vi "ReadFromFIFO.vi"(10 "stop":bool) -> (2 "This is what I told you!":string)   [LabVIEW 2011]
doc: "Elizabeth Mahon\nBased off of example from LabView and IGVC 3.2.1 Read VectorNav.\nReads data from compass sensor on port 1 of the serial module from a FIFO and outputs it as a string.\nStarts as waiting, then when it reads $ (first element of compass string) starts reading and adds everything it reads together until it reaches *ss (where ss can be anything, the \"two digit checksum\"), and then stops and outputs the string.\nOnly reads the string once - must be run in a while loop for multiple readings.\nJust shuts down if it has an error. In the future, we might want to output if it has an error."
uses:
  <vilib>/FPGAPlugInAG/cRIO-9113/niLvFpga_Open_cRIO-9113.vi
  <vilib>/rvi/interface/common/dynamic/niFpgaDynamicAddResources.vi
  <vilib>/Utility/error.llb/Error Cluster From Error Code.vi
  <vilib>/rvi/errors/niLvFpgaAdjustHostInterfaceError.vi
  <vilib>/FPGAPlugInAG/Dynamic/niLvFpga_Close_Dynamic.vi
  <vilib>/rvi/interface/nirviOpenFPGA/nirviOpenFPGA.xnode
  FPGA Bitfiles/SailBot_FPGATarget_WriteToFIFO_EBA82491.lvbitx
  1A-FPGA/1A Code/WriteToFIFO.vi
  <vilib>/rvi/interface/nirviMethod/nirviMethod.xnode
  <vilib>/rvi/interface/nirviCloseFPGA/nirviCloseFPGA.xnode
  <vilib>/FPGAPlugInAG/Dynamic/niLvFpga_ReadFifo_Dynamic.vi
  <vilib>/rvi/errors/niLvFpgaMergeErrorWithErrorCode.vi
panel:
  out "Current Status":enum16{"Waiting", "Reading", "Time Out!"}(ring)
  out "Data":i16[](array[numeric])
  in  "Status":enum16{"Waiting", "Reading", "Time Out!"}(ring)
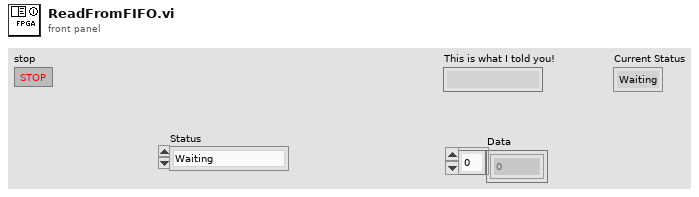
[diagram p1: front panel]
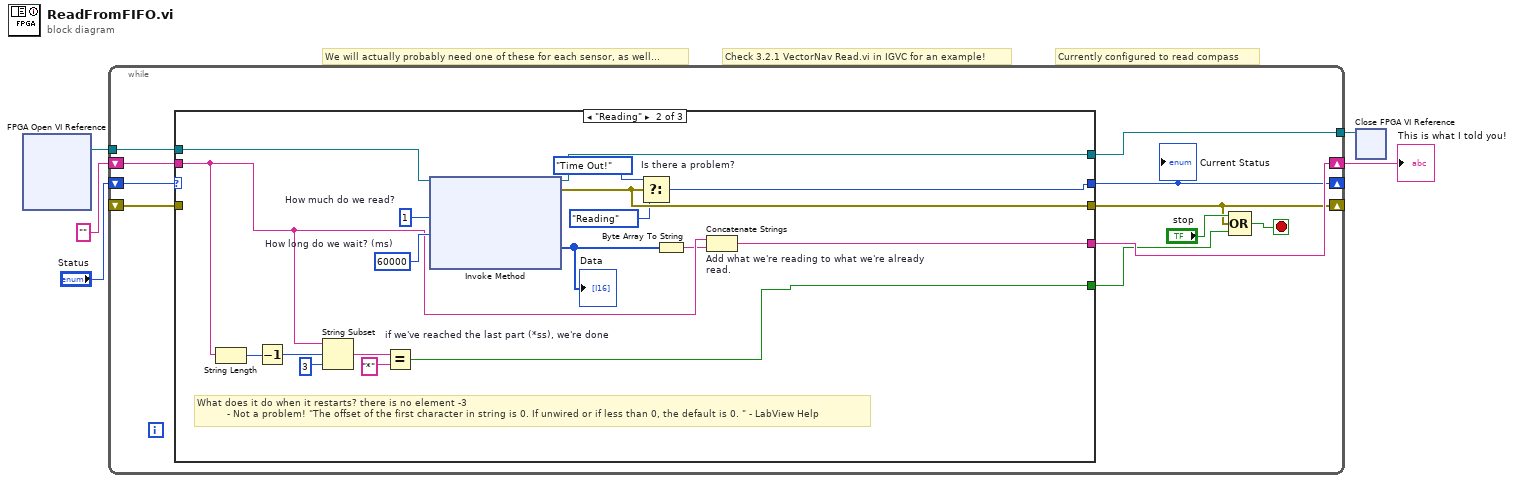
[diagram p0: block diagram]
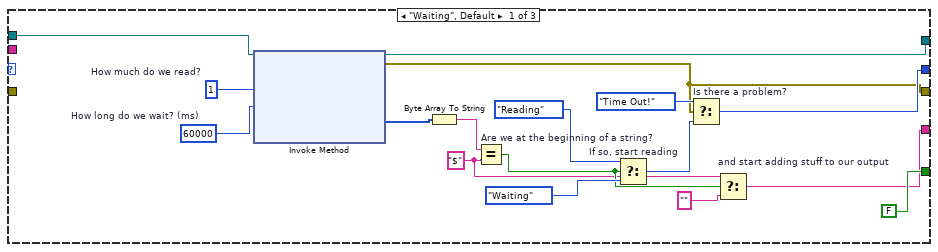
[diagram p2: hidden frame]
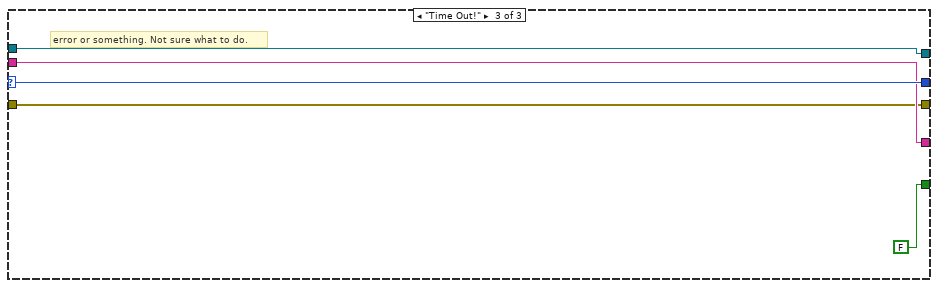
[diagram p3: hidden frame]
diagram:
  # "Currently configured to read compass"
  # "Check 3.2.1 VectorNav Read.vi in IGVC for an example!"
  # "We will actually probably need one of these for each sensor, as well..."
  n1 = xnode "FPGA Open VI Reference"() -> ("FPGA VI Reference Out"=w5:refnum<k20>)  [unwired: 2 in, 1 out]
  n2 = while {
    tunnel: w5 -> [w16]
    shift-right: [w14] -> w4
    shift-left: "" -> [w15]
    shift-right: [w6] -> _
    shift-left: "Status" -> [w13]
    shift-right: [w10] -> _
    shift-left: _ -> [w9]
    tunnel: [w7] -> w1
    stop <- w11 stop-if-true
    n3 = case shown="\"Reading\"" w13 {
      selector: w13 -> [_ _ w56]
      tunnel: w16 -> [w33 w49 w52]
      tunnel: w15 -> [_ w39 w55]
      tunnel: [w19 w45 w55] -> w14
      tunnel: [w24 w47 w56] -> w6
      tunnel: [w23 w46 w54] -> w10
      tunnel: w9 -> [_ _ w54]
      tunnel: [FALSE w36 FALSE] -> w8
      tunnel: [w32 w37 w52] -> w7
      frame "Waiting", Default {
        w18 = "$" ("x")
        w30 = 60000  # How long do we wait? (ms)
        w31 = u32 1  # How much do we read?
        n4 = xnode "Invoke Method"("FPGA VI Reference In"=w33, "Number of Elements"=w31, "Timeout (ms)"=w30) -> ("FPGA VI Reference Out"=w32:refnum<k20>, "error out"=w23:errorcluster, "Data"=w29:i16[])  [unwired: 1 in, 1 out]
        n5 = Byte Array To String(unsigned byte array=w29) -> (string=w17:string)
        n6 = Equal? "Are we at the beginning of a string?"(x=w17, y=w18) -> (x = y?=w20:bool)
        n7 = Select "If so, start reading"(t=enum16{"Waiting", "Reading", "Time Out!"}."Reading", s=w20, f=enum16{"Waiting", "Reading", "Time Out!"}."Waiting" ("Current Status")) -> (s? t:f=w26:enum16{"Waiting", "Reading", "Time Out!"})
        n8 = Select "Is there a problem?"(t=enum16{"Waiting", "Reading", "Time Out!"}."Time Out!", s=w23, f=w26) -> (s? t:f=w24:enum16{"Waiting", "Reading", "Time Out!"})
        n9 = Select "and start adding stuff to our output"(t=w18, s=w20, f="") -> (s? t:f=w19:string)
      }
      frame "Reading" {
        w50 = 60000  # How long do we wait? (ms)
        w51 = u32 1  # How much do we read?
        # "What does it do when it restarts? there is no element -3\n          - Not a problem! \"The offset of the first character in string is 0. If unwired or if less than 0, the default is 0. \" - LabView Help"
        n10 = String Length(string=w39) -> (length=w44:i32)
        n11 = Decrement(x=w44) -> (x-1=w43:i32)
        n12 = String Subset(string=w39, offset (0)=w43, length (rest)=3 ("length (rest)")) -> (substring=w41:string)
        n13 = Equal? "if we've reached the last part (*ss), we're done"(x=w41, y="*") -> (x = y?=w36:bool)
        n14 = xnode "Invoke Method"("FPGA VI Reference In"=w49, "Number of Elements"=w51, "Timeout (ms)"=w50) -> ("FPGA VI Reference Out"=w37:refnum<k20>, "error out"=w46:errorcluster, "Data"=w48:i16[])  [unwired: 1 in, 1 out]
        "Data" <- w48
        n15 = Select "Is there a problem?"(t=enum16{"Waiting", "Reading", "Time Out!"}."Time Out!", s=w46, f=enum16{"Waiting", "Reading", "Time Out!"}."Reading" ("Status")) -> (s? t:f=w47:enum16{"Waiting", "Reading", "Time Out!"})
        n16 = Byte Array To String(unsigned byte array=w48) -> (string=w38:string)
        n17 = Concatenate Strings "Add what we're reading to what we're already read."(w39, w38) -> (w45:string)
      }
      frame "Time Out!" {
        # "error or something. Not sure what to do."
      }
    }
    "Current Status" <- w6
    n18 = Compound Arithmetic op=OR("stop", w10, w8) -> (w11:bool)
  }
  "This is what I told you!" <- w4
  n19 = xnode "Close FPGA VI Reference"("FPGA VI Reference In"=w1) -> ()  [unwired: 1 in, 1 out]
